vi "IS Send.vi"(8 "error in (no error)":errorcluster, 9 "JSON Custer Array in":T1[](array[typedef]), 10 "IS Bucket Session":T2, 11 "IS Session in":T3) -> (0 "Error out":errorcluster, 1 "Response Body":string, 2 "IS Bucket Session out":T2, 3 "IS Session out":T3, 4 "Rate Limit Reached?":bool, 5 "Response Headers":string)   [LabVIEW 2013]
uses:
  <vilib>/httpClient/LabVIEWHTTPClient.lvlib
  <vilib>/httpClient/POSTBuffer.vi
  Custom Data Types/IS Bucket Session.ctl
  <vilib>/httpClient/ClientHandle.ctl
  Custom Data Types/IS Session.ctl
  Custom Data Types/IS Data Point TypeDef (String).ctl
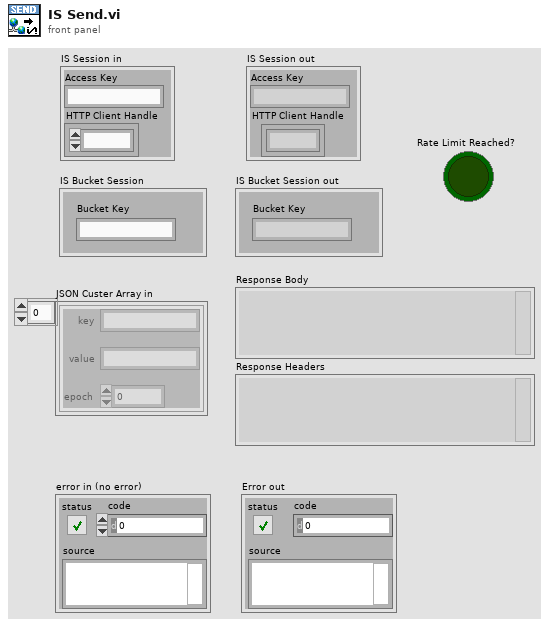
[diagram p1: front panel]
types:
  T1 = typedef "IS Data Point TypeDef (String).ctl" = cluster{"key":string, "value":string, "epoch":dbl}
  T2 = typedef "IS Bucket Session.ctl" = cluster{"Bucket Key":string}
  T3 = typedef "IS Session.ctl" = cluster{"Access Key":string, "HTTP Client Handle":T4}
  T4 = typedef "LabVIEWHTTPClient.lvlib/ClientHandle.ctl" = refnum<k1>
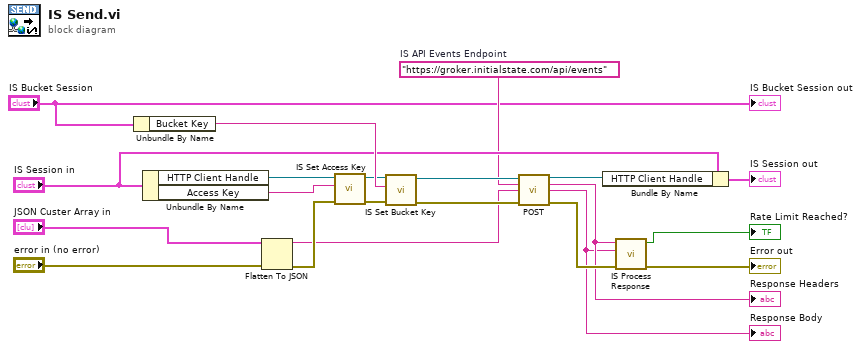
[diagram p0: block diagram]
diagram:
  w14 = "https://groker.initialstate.com/api/events"  # IS API Events Endpoint
  n1 = Unbundle By Name("IS Bucket Session") -> ("Bucket Key"=w21:string)
  n2 = Unbundle By Name("IS Session in") -> ("HTTP Client Handle"=w12:T4, "Access Key"=w13:string)
  n3 = Flatten To JSON(anything="JSON Custer Array in", error in (no error)="error in (no error)") -> (JSON string=w6:string, 11:w7:errorcluster)  [unwired: 1 in]
  n4 = call "IS Set Access Key.vi"("HTTP Client Handle in"=w12, "Access Key"=w13, "error in (no error)"=w7) -> ("HTTP Client Handle out"=w18:T4, "error out"=w19:errorcluster)  [unwired: 6 in]
  n5 = call "IS Set Bucket Key.vi"("HTTP Client Handle in"=w18, "Bucket Key"=w21, "error in (no error)"=w19) -> ("HTTP Client Handle out"=w20:T4, "error out"=w10:errorcluster)  [unwired: 6 in]
  n6 = call-poly <vilib>:"POST.vi"("client handle"=w20, "url"=w14, "buffer"=w6, "error in (no error)"=w10) -> ("client handle out"=w16:T4, "headers"=w4:string, "body"=w3:string, "error out"=w5:errorcluster)  [unwired: 8 in]
  "Response Body" <- w3
  "Response Headers" <- w4
  n7 = Bundle By Name(cluster="IS Session in", "HTTP Client Handle"=w16) -> (→"IS Session out":T3)
  n8 = call "IS Process Response.vi"("error in (no error)"=w5, "Response Body"=w3, "Response Headers"=w4) -> ("error in (no error) 2"=→"Error out":errorcluster, "Rate Limit Reached"=→"Rate Limit Reached?":bool)  [unwired: 7 in]
  "IS Bucket Session out" <- "IS Bucket Session"
